vi "Write Light Settings.vi"(8 "error in (no error)":errorcluster, 10 "Light Settings":T1, 11 "Supervisor in":refnum<class "Supervisor.lvclass">) -> (0 "error out":errorcluster, 3 "Supervisor out":refnum<class "Supervisor.lvclass">)   [LabVIEW 2014, in "Supervisor.lvclass"]
uses:
  Supervisor.lvclass
  Supervisor.lvclass/Supervisor.ctl
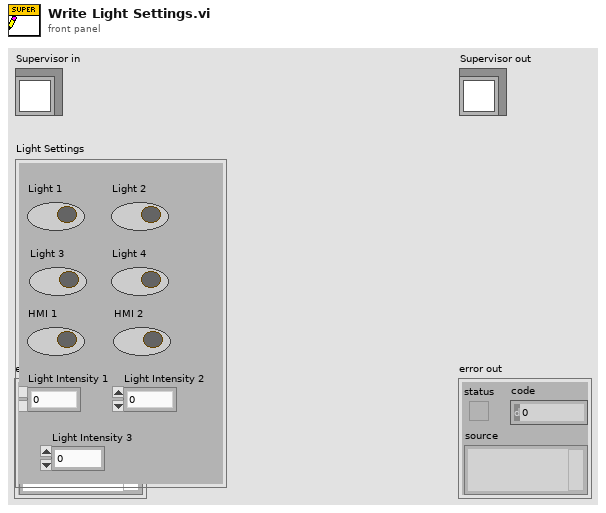
[diagram p1: front panel]
types:
  T1 = cluster{"Light 1":bool, "Light 2":bool, "Light 3":bool, "Light 4":bool, "HMI 1":bool, "HMI 2":bool, "Light Intensity 1":i32, "Light Intensity 2":i32, "Light Intensity 3":i8}
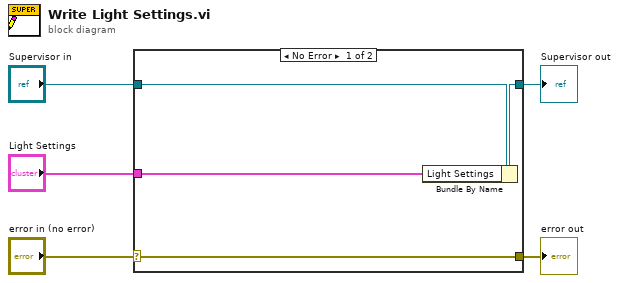
[diagram p0: block diagram]
diagram:
  n1 = case shown="No Error" "error in (no error)" {
    selector: "error in (no error)" -> [w9 w10]
    tunnel: [w9 w10] -> w4
    tunnel: [w7 w11] -> w2
    tunnel: "Supervisor in" -> [w8 w11]
    tunnel: "Light Settings" -> [w6 _]
    frame No Error {
      n2 = Bundle By Name(cluster=w8, "Light Settings"=w6) -> (w7:refnum<class "Supervisor.lvclass">)
    }
    frame Error {
    }
  }
  "error out" <- w4
  "Supervisor out" <- w2
